vi "Test Show Chars Missing and Added.vi"(11 "Test Case In":refnum<class "Diff Tool Test.lvclass">) -> (0 "error out":errorcluster, 3 "Test Case Out":refnum<class "Diff Tool Test.lvclass">)   [LabVIEW 2020, in "Diff Tool Test.lvclass"]
uses:
  Diff Tool Test.lvclass
  usr/local/natinst/LabVIEW-2026-64/vi.lib/Astemes/LUnit/Test Case.lvclass
  <vilib>/Astemes/LUnit/Test Case.lvclass/Test Case.ctl
  4993e8ee-a06a-463a-9684-69129f64d5ce.vi
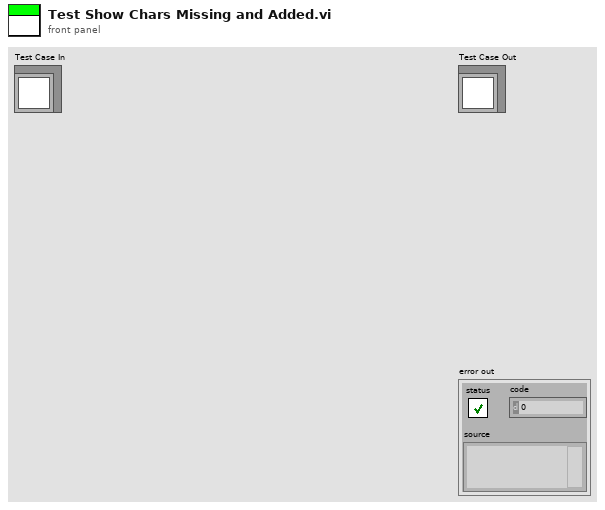
[diagram p1: front panel]
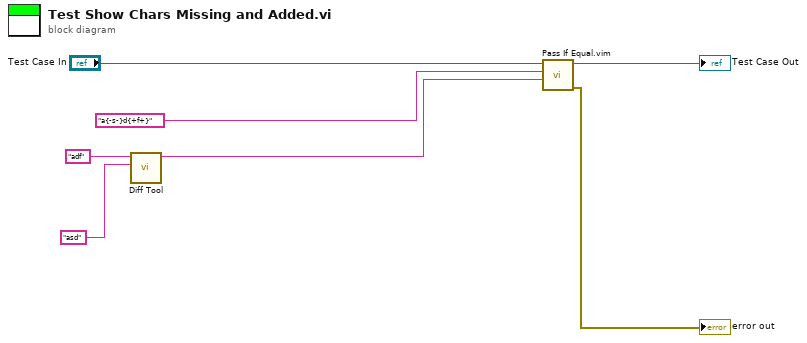
[diagram p0: block diagram]
diagram:
  n1 = call "Diff Tool.vi"("Reference"="asd" ("Target"), "Target"="adf" ("Reference")) -> ("Result"=w2:string)  [unwired: 8 in, 1 out]
  n2 = call "Pass If Equal.vim"("Actual"=w2, "Expected"="a{-s-}d{+f+}" ("Reference"), "LUnit Test Case In"="Test Case In") -> ("error out"=→"error out":errorcluster, "LUnit Test Case Out"=→"Test Case Out":refnum<class "Diff Tool Test.lvclass">)  [unwired: 7 in]
